vi "IC_SoftwareTrigger.vi"(1 "ICImagingControl 3":refnum<k7>) -> (0 "ICImagingControl 2":refnum<k7>)   [LabVIEW 2015]
doc: "This VI performs an software trigger push for The Imaging Source cameras."
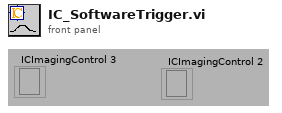
[diagram p1: front panel]
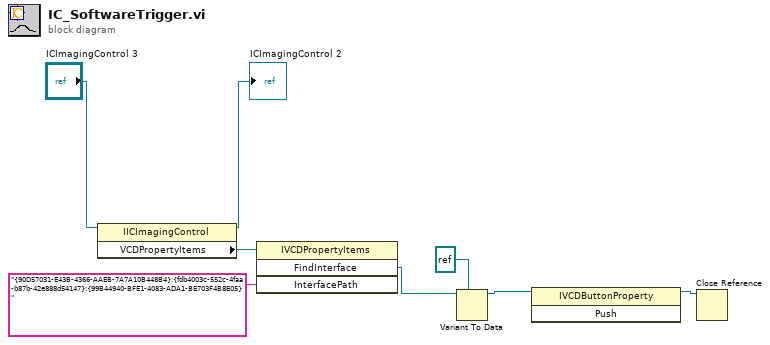
[diagram p0: block diagram]
diagram:
  n1 = property class="IICImagingControl"(reference="ICImagingControl 3") -> (reference out=→"ICImagingControl 2":refnum<k7>, "VCDPropertyItems"=w3:refnum<k7>)  [unwired: 1 in, 1 out]
  n2 = invoke class="IVCDPropertyItems" method="FindInterface"(reference=w3, "InterfacePath"="{90D57031-E43B-4366-AAEB-7A7A10B448B4}:{fdb4003c-552c-4faa-b87b-42e888d54147}:{99B44940-BFE1-4083-ADA1-BE703F4B8E05}") -> ("FindInterface"=w5:refnum<k7>)  [unwired: 2 in, 3 out]
  n3 = Variant To Data(type=refnum<k7> refnum ("ICImagingControl3.IVCDButtonProperty"), Variant=w5) -> (data=w7:refnum<k7>)  [unwired: 1 in, 1 out]
  n4 = invoke class="IVCDButtonProperty" method="Push"(reference=w7) -> (reference out=w8:refnum<k7>)  [unwired: 2 in, 2 out]
  n5 = Close Reference(reference=w8) -> ()  [unwired: 1 in, 1 out]
